vi "Array Pointer.vi"(8 "error in (no error)":errorcluster caption="错误输入（无错误）", 10 "Size":i32=8, 11 "Reset":bool) -> (0 "error out":errorcluster caption="错误输出", 1 "Full":bool, 2 "Pre Pos":i32, 3 "Current Pos":i32)   [LabVIEW 2012]
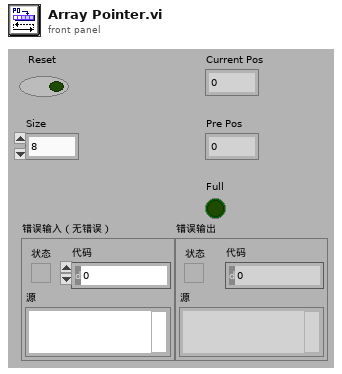
[diagram p1: front panel]
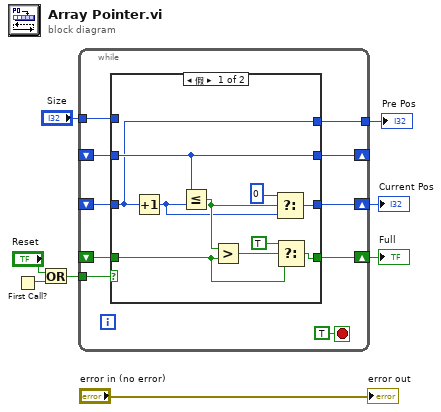
[diagram p0: block diagram]
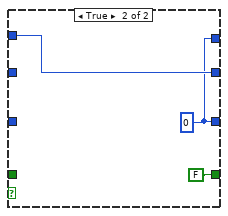
[diagram p2: hidden frame]
diagram:
  n1 = First Call?() -> (First Call?: T/F=w7:bool)
  n2 = Or(x="Reset", y=w7) -> (x .or. y?=w6:bool)
  n3 = while {
    tunnel: w6 -> [w17]
    shift-right: [w16] -> w2
    shift-left: _ -> [w10]
    shift-right: [w15] -> w5
    shift-left: _ -> [w11]
    shift-right: [w13] -> _
    shift-left: _ -> [w12]
    tunnel: "Size" -> [w14]
    tunnel: [w9] -> w3
    stop <- TRUE stop-if-true
    n4 = case shown="假" w17 {
      tunnel: [w25 FALSE ("Full")] -> w16
      tunnel: [w23 w29] -> w15
      tunnel: w14 -> [_ w30]
      tunnel: [w28 w30] -> w13
      tunnel: w12 -> [w28 _]
      tunnel: w11 -> [w20 _]
      tunnel: w10 -> [w22 _]
      tunnel: [w20 w29] -> w9
      frame False {
        n5 = Increment(x=w20) -> (x+1=w19:i32)
        n6 = Less Or Equal?(x=w28, y=w19) -> (x <= y?=w21:bool)
        n7 = Greater?(x=w21, y=w22) -> (0:w27:bool)
        n8 = Select(t=0 ("Pointer"), s=w21, f=w19) -> (s? t:f=w23:i32)
        n9 = Select(t=TRUE ("Full"), s=w27, f=w22) -> (s? t:f=w25:bool)
      }
      frame True {
        w29 = 0 ("Pointer")
      }
    }
  }
  "Current Pos" <- w5
  "Full" <- w2
  "Pre Pos" <- w3
  "error out" <- "error in (no error)"
